vi "sub vi - AI USB4704 (3)  Create Task v1.vi"(0 "Task In 0":dbl, 5 "Task In 1":dbl, 7 "Task In 2":dbl) -> (4 "TASK USB 0":i32, 6 "TASK USB 1":i32, 8 "TASK USB 2":i32, 14 "AI Task Er":bool, 15 "error array":errorcluster[](array[cluster]))   [LabVIEW 2013]
uses:
  program files/Global 1.vi
  <userlib>/DAQNavi Polymorphic VI/create/DAQNavi Create Channel(AI-Voltage).vi
  <userlib>/DAQNavi Polymorphic VI/configure/timing/DAQNavi Timing(Convert Clock).vi
  <userlib>/DAQNavi Polymorphic VI/configure/DAQNavi Get Property/AI/DAQNaviGet_AI_ConvertClock_Rate.vi
panel:
  in  "RATE(Hz)":dbl
  in  "Tab Control":enum32{"Tasks In", "USB #0", "USB #1", "USB #2"}(tab)
  out "physical channels 0":string="DemoDevice,BID#0/ai0:1" caption="property value"
  out "value range 0":string="+/- 5 V" caption="property value"
  out "convert rate 0":dbl
  out "physical channels 1":string="DemoDevice,BID#0/ai0:1" caption="property value"
  out "value range  1":string="+/- 5 V" caption="property value"
  out "convert rate 1":dbl
  out "physical channels 2":string="DemoDevice,BID#0/ai0:1" caption="property value"
  out "value range  2":string="+/- 5 V" caption="property value"
  out "convert rate 2":dbl
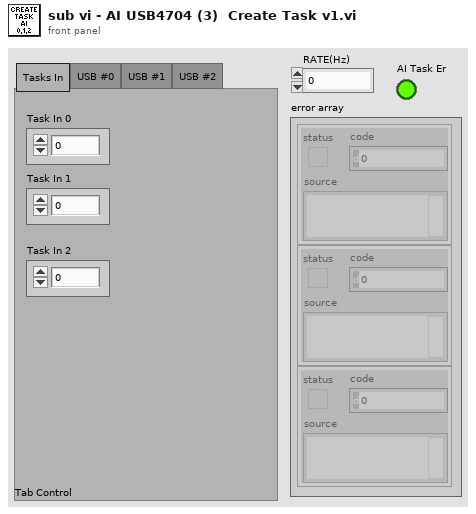
[diagram p1: front panel]
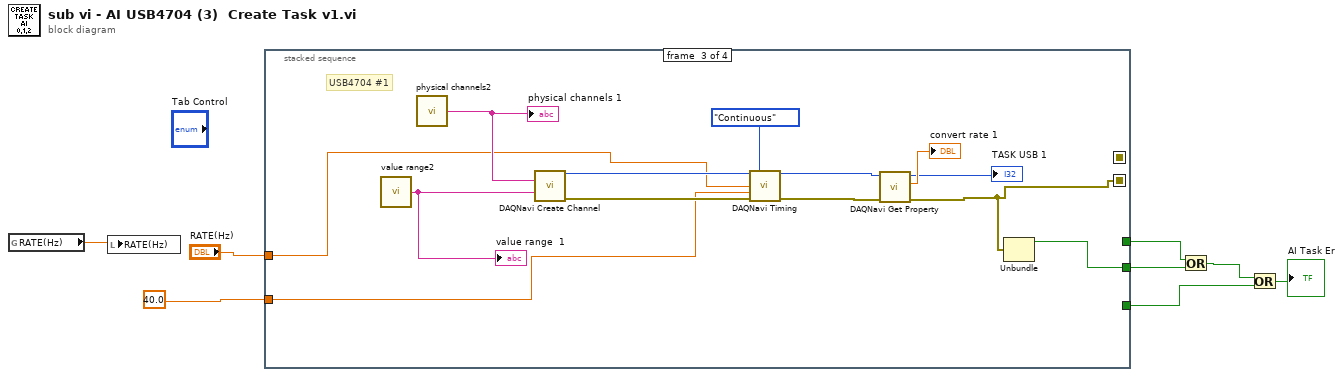
[diagram p0: block diagram]
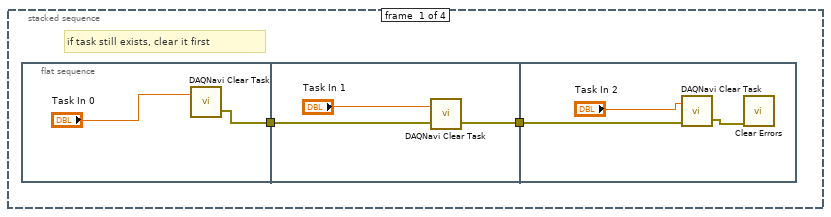
[diagram p2: hidden frame]
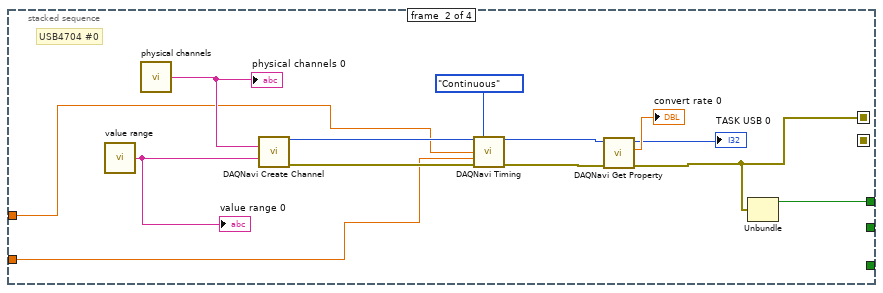
[diagram p3: hidden frame]
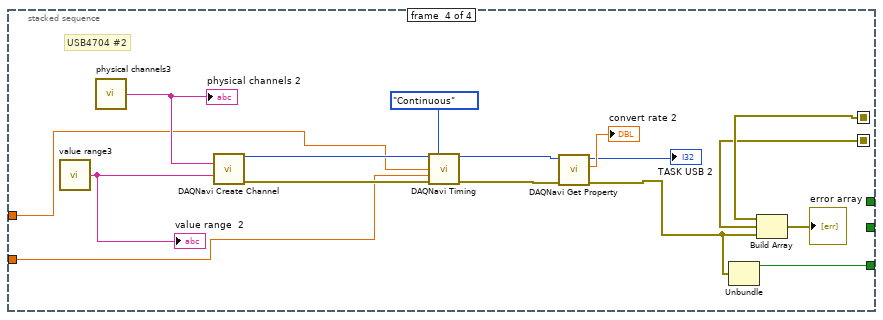
[diagram p4: hidden frame]
diagram:
  n1 = global read "Global 1.vi" "RATE(Hz)"() -> (w7:dbl)
  n2 = local write "RATE(Hz)"(w7) -> ()
  n3 = stacked-sequence {
    seq-local: [_ w20 _ _] -> [_ _ _ w51]
    seq-local: [_ _ w33 _] -> [_ _ _ w50]
    tunnel: "RATE(Hz)" -> [_ w22 w35 w48]
    tunnel: 40.0 -> [_ w21 w34 w47]
    tunnel: [_ _ _ w45] -> w3
    tunnel: [_ w19 _ _] -> w2
    tunnel: [_ _ w32 _] -> w1
    frame #0 {
      # "if task still exists, clear it first"
      n4 = flat-sequence {
        tunnel: [w12] -> w10
        tunnel: w10 -> [w15]
        tunnel: [w14] -> w9
        tunnel: w9 -> [w18]
        frame #0 {
          n5 = call <userlib>:"DAQNavi Clear Task.vi"("task in"="Task In 0") -> ("error out"=w12:errorcluster)  [unwired: 2 in]
        }
        frame #1 {
          n6 = call <userlib>:"DAQNavi Clear Task.vi"("error in (no error)"=w15, "task in"="Task In 1") -> ("error out"=w14:errorcluster)  [unwired: 1 in]
        }
        frame #2 {
          n7 = call <userlib>:"DAQNavi Clear Task.vi"("error in (no error)"=w18, "task in"="Task In 2") -> ("error out"=w17:errorcluster)  [unwired: 1 in]
          n8 = call <vilib>:"Clear Errors.vi"("error in (no error)"=w17) -> ()  [unwired: 6 in, 1 out]
        }
      }
    }
    frame #1 {
      # "USB4704 #0"
      n9 = call "value range"() -> ("property value"=w31:string)  [unwired: 1 out]
      "value range 0" <- w31
      n10 = call "physical channels"() -> ("property value"=w30:string)  [unwired: 1 out]
      "physical channels 0" <- w30
      n11 = call-poly <userlib>:"DAQNavi Create Channel.vi"("physical channels"=w30, "value range"=w31) -> ("task out"=w24:i32, "error out"=w25:errorcluster)  [unwired: 3 in, 9 out]
      n12 = call-poly <userlib>:"DAQNavi Timing.vi"("task in"=w24, "sample mode"=enum16{"Finite", "Continuous"}."Continuous", "rate"=w22, "samples per channel"=w21, "error in (no error)"=w25) -> ("task out"=w27:i32, "error out"=w28:errorcluster)  [unwired: 1 in, 8 out]
      n13 = call-poly <userlib>:"DAQNavi Get Property.vi"("error in (no error)"=w28, "task in"=w27) -> ("error out"=w20:errorcluster, "rate"=→"convert rate 0":dbl, "task out"=→"TASK USB 0":i32)  [unwired: 7 out]
      n14 = Unbundle(w20) -> ("status"=w19:bool)  [unwired: 2 out]
    }
    frame #2 {
      # "USB4704 #1"
      n15 = call "value range2"() -> ("property value"=w44:string)  [unwired: 1 out]
      "value range  1" <- w44
      n16 = call "physical channels2"() -> ("property value"=w43:string)  [unwired: 1 out]
      "physical channels 1" <- w43
      n17 = call-poly <userlib>:"DAQNavi Create Channel.vi"("physical channels"=w43, "value range"=w44) -> ("task out"=w37:i32, "error out"=w38:errorcluster)  [unwired: 3 in, 9 out]
      n18 = call-poly <userlib>:"DAQNavi Timing.vi"("task in"=w37, "sample mode"=enum16{"Finite", "Continuous"}."Continuous", "rate"=w35, "samples per channel"=w34, "error in (no error)"=w38) -> ("task out"=w40:i32, "error out"=w41:errorcluster)  [unwired: 1 in, 8 out]
      n19 = call-poly <userlib>:"DAQNavi Get Property.vi"("error in (no error)"=w41, "task in"=w40) -> ("error out"=w33:errorcluster, "rate"=→"convert rate 1":dbl, "task out"=→"TASK USB 1":i32)  [unwired: 7 out]
      n20 = Unbundle(w33) -> ("status"=w32:bool)  [unwired: 2 out]
    }
    frame #3 {
      # "USB4704 #2"
      n21 = call "value range3"() -> ("property value"=w60:string)  [unwired: 1 out]
      "value range  2" <- w60
      n22 = call "physical channels3"() -> ("property value"=w59:string)  [unwired: 1 out]
      "physical channels 2" <- w59
      n23 = call-poly <userlib>:"DAQNavi Create Channel.vi"("physical channels"=w59, "value range"=w60) -> ("task out"=w53:i32, "error out"=w54:errorcluster)  [unwired: 3 in, 9 out]
      n24 = call-poly <userlib>:"DAQNavi Timing.vi"("task in"=w53, "sample mode"=enum16{"Finite", "Continuous"}."Continuous", "rate"=w48, "samples per channel"=w47, "error in (no error)"=w54) -> ("task out"=w56:i32, "error out"=w57:errorcluster)  [unwired: 1 in, 8 out]
      n25 = call-poly <userlib>:"DAQNavi Get Property.vi"("error in (no error)"=w57, "task in"=w56) -> ("error out"=w46:errorcluster, "rate"=→"convert rate 2":dbl, "task out"=→"TASK USB 2":i32)  [unwired: 7 out]
      n26 = Unbundle(w46) -> ("status"=w45:bool)  [unwired: 2 out]
      n27 = Build Array(w51, w50, w46) -> (→"error array":errorcluster[])
    }
  }
  n28 = Or(x=w2, y=w1) -> (x .or. y?=w4:bool)
  n29 = Or(x=w4, y=w3) -> (x .or. y?=→"AI Task Er":bool)
